vi "Hide Splash.vi"(8 "error in (no error)":errorcluster, 11 "Basic Splash in":refnum<class "Basic Splash.lvclass">) -> (0 "error out":errorcluster, 3 "Basic Splash out":refnum<class "Basic Splash.lvclass">)   [LabVIEW 2020, in "Volatus.lvlib" / "Basic Splash.lvclass"]
uses:
  Basic Splash.lvclass
  Basic Splash.lvclass/Basic Splash.ctl
  Event Type.ctl
  Event Data.ctl
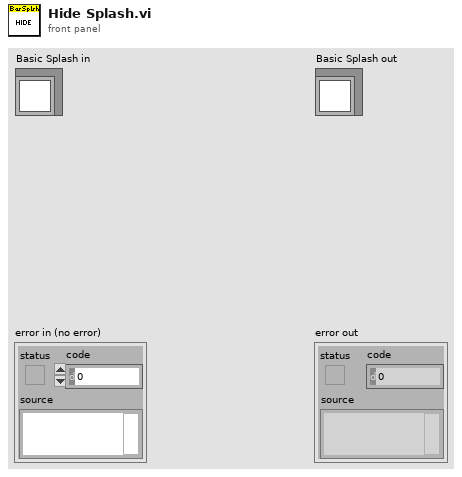
[diagram p1: front panel]
types:
  T1 = typedef "Volatus.lvlib/Basic Splash.lvclass/Event Data.ctl" = cluster{"Type":T2, "Status":string}
  T2 = typedef "Volatus.lvlib/Basic Splash.lvclass/Event Type.ctl" = enum16{"Show", "Hide", "Update", "Close"}
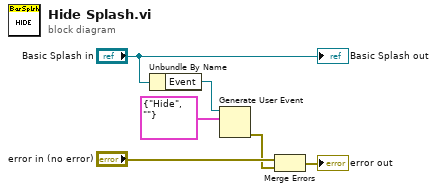
[diagram p0: block diagram]
diagram:
  n1 = Unbundle By Name("Basic Splash in") -> ("Event"=w4:refnum<user-event>)
  n2 = Generate User Event(user event=w4, event data cluster=T1 {"Type"=enum."Hide", "Status"=""} ("event data")) -> (error out=w1:errorcluster)  [unwired: 2 in, 1 out]
  n3 = Merge Errors("error in (no error)", w1) -> (→"error out":errorcluster)
  "Basic Splash out" <- "Basic Splash in"
